vi "New Error Cluster (Custom).vi"(7 "size":i32 format="%d bytes", 9 "class name (\"\")":string, 10 "library name (\"\")":string, 11 "vi name (\"\")":string) -> (1 "initial offset":i32, 3 "error out":errorcluster)   [LabVIEW 2027, in "Static Errors.lvlib"]
doc: "Returns an error cluster with an allocated source buffer of the specified <b>size</b> in bytes. The minimum size is 9 bytes, required by other data fields in the error cluster."
uses:
  Static Errors.lvlib
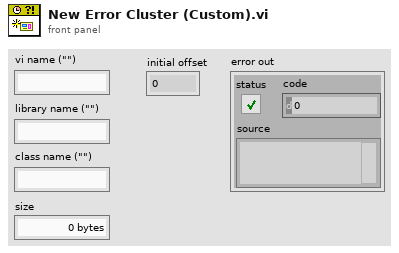
[diagram p1: front panel]
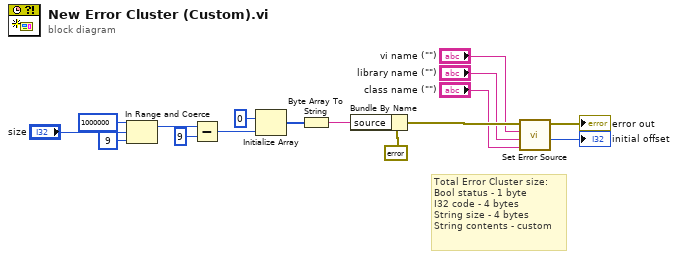
[diagram p0: block diagram]
diagram:
  # "Total Error Cluster size:\nBool status - 1 byte\nI32 code - 4 bytes\nString size - 4 bytes\nString contents - custom"
  n1 = In Range and Coerce(upper limit=1000000, x="size", lower limit=9) -> (coerced(x)=w12:i32)  [unwired: 1 out]
  n2 = Subtract(x=w12, y=9) -> (x-y=w10:i32)
  n3 = Initialize Array(u8 0 ("element"), w10) -> (w8:u8[])
  n4 = Byte Array To String(unsigned byte array=w8) -> (string=w7:string)
  n5 = Bundle By Name(cluster=errorcluster {"status"=FALSE, "code"=0, "source"=""} ("error in (no error)"), "source"=w7) -> (w6:errorcluster)
  n6 = call "Set Error Source.vi"("class name (\"\")"="class name (\"\")", "library name (\"\")"="library name (\"\")", "vi name"="vi name (\"\")", "error in"=w6) -> ("initial offset"=→"initial offset":i32, "error out"=→"error out":errorcluster)  [unwired: 6 in]
